vi "Merge Records.vi"(4 "Records":dbl[][][](array[numeric])) -> (1 "Channel Data":dbl[][](array[numeric]))   [LabVIEW 2013]
panel:
  out "size(s) 2":i32[](array[numeric])
  out "size(s)":i32[](array[numeric])
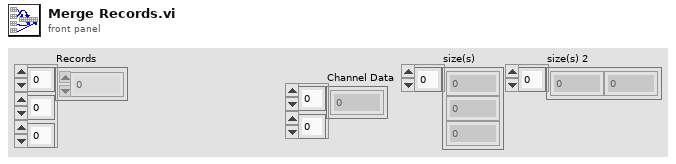
[diagram p1: front panel]
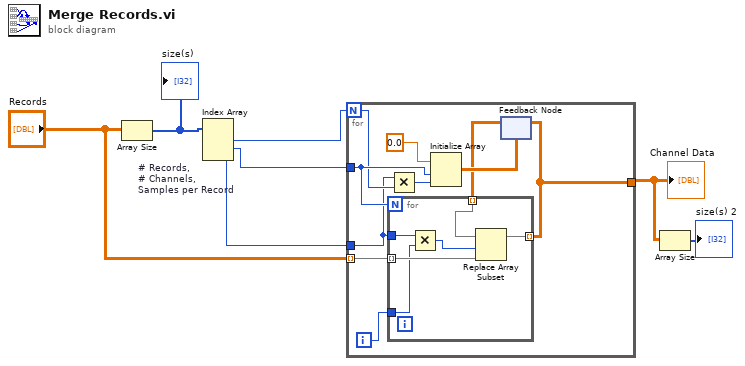
[diagram p0: block diagram]
diagram:
  n1 = Array Size(array="Records") -> (size(s)=w6:i32[])
  "size(s)" <- w6
  n2 = Index Array "# Records,\n# Channels,\nSamples per Record"(array=w6) -> (element #1=w5:i32, element #2=w4:i32, element #3=w3:i32)  [unwired: 3 in]
  n3 = for {
    N: w5 -> [w13]
    tunnel: "Records" -> [w17] mode=indexing
    tunnel: w4 -> [w14]
    tunnel: w3 -> [w11]
    tunnel: [w8] -> w2
    i -> [w10]
    n4 = Multiply(x=w11, y=w13) -> (x*y=w15:i32)
    n5 = Initialize Array(0.0 ("element"), w14, w15) -> (w12:dbl[][])
    n6 = feedback #1(w12) -> (w9:dbl[][])
    n7 = for {
      N: w14 -> [_]
      tunnel: w17 -> [w22] mode=indexing
      tunnel: w9 -> [w23] mode=indexing
      tunnel: w11 -> [w21]
      tunnel: w10 -> [w20]
      tunnel: [w18] -> w8 mode=indexing
      n8 = Multiply(x=w21, y=w20) -> (x*y=w19:i32)
      n9 = Replace Array Subset(array=w23, new element=w22, index=w19) -> (w18:dbl[])
    }
    n10 = feedback-in #1(w8) -> ()
  }
  "Channel Data" <- w2
  n11 = Array Size(array=w2) -> (size(s)=→"size(s) 2":i32[])
